vi "Run.vi"(8 "error in (no error)":errorcluster, 9 "s on last turn":dbl, 10 "Maze (0: Empty, -1: Enemy. >0: Teammate":i32[][](array[numeric]), 11 "Spawn in":refnum<class "Spawn.lvclass">) -> (0 "error out":errorcluster, 1 "Direction":T1, 2 "Action":T2, 3 "Spawn out":refnum<class "Spawn.lvclass">, 4 "Replicated":refnum<class "Runner.lvclass">)   [LabVIEW 2014, in "Spawn.lvclass"]
uses:
  Spawn.lvclass
  Action Enum.ctl
  Direction Enum.ctl
  Runner.lvclass
  Spawn.lvclass/Spawn.ctl
  Attack/Attack.lvclass
  Attack/Attack.lvclass/Attack.ctl
  Attack/Write Deviation.vi
  Attack/Write Direction.vi
  Attack/Write Frequency.vi
  SquareBattle.lvclass
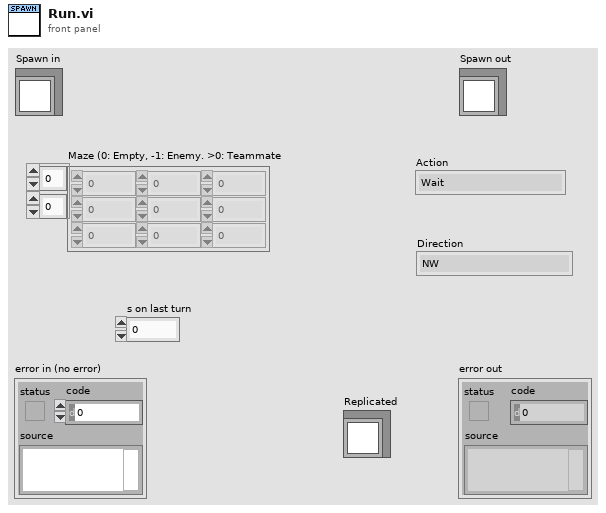
[diagram p1: front panel]
types:
  T1 = typedef "SquareBattle.lvclass/Direction Enum.ctl" = enum16{"NW", "N", "NE", "E", "SE", "S", "SW", "W"}
  T2 = typedef "SquareBattle.lvclass/Action Enum.ctl" = enum16{"Wait", "Move", "Attack", "Replicate"}
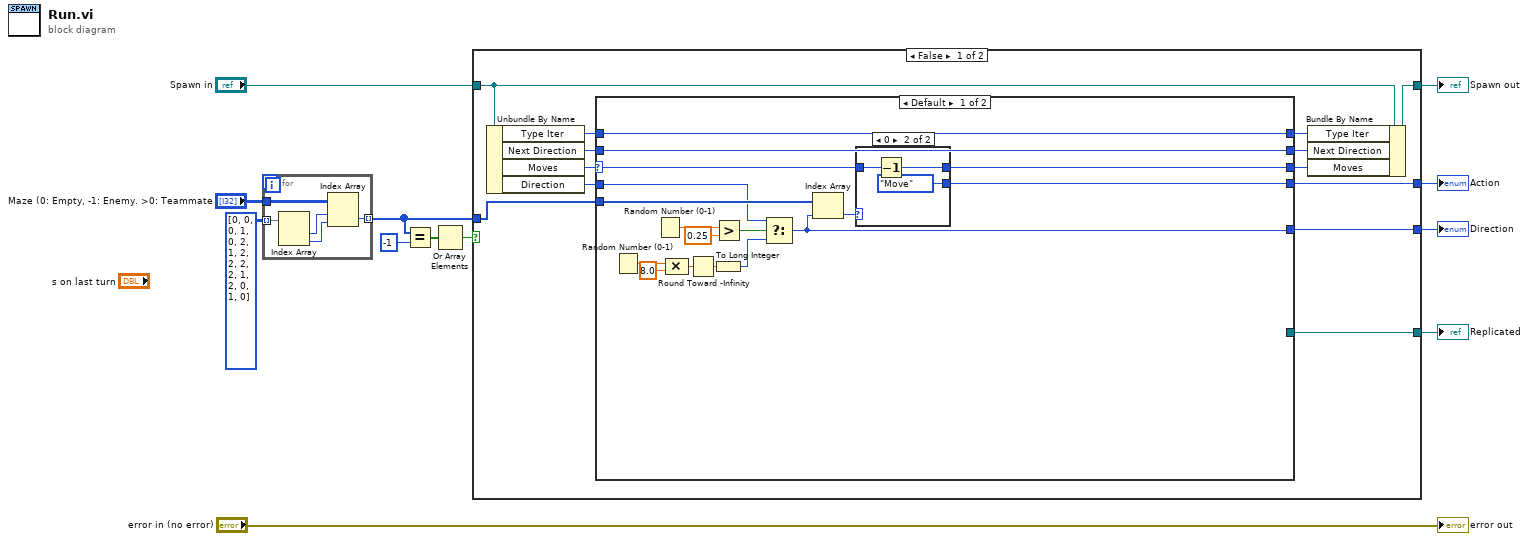
[diagram p0: block diagram]
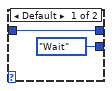
[diagram p2: hidden frame]
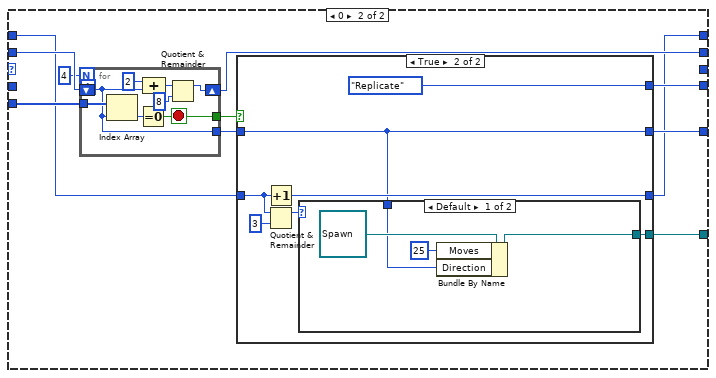
[diagram p3: hidden frame]
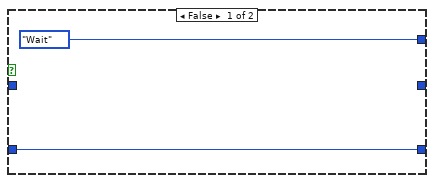
[diagram p4: hidden frame]
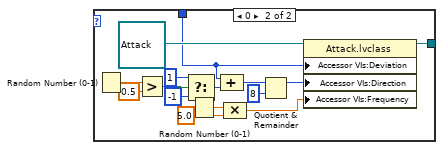
[diagram p5: hidden frame]
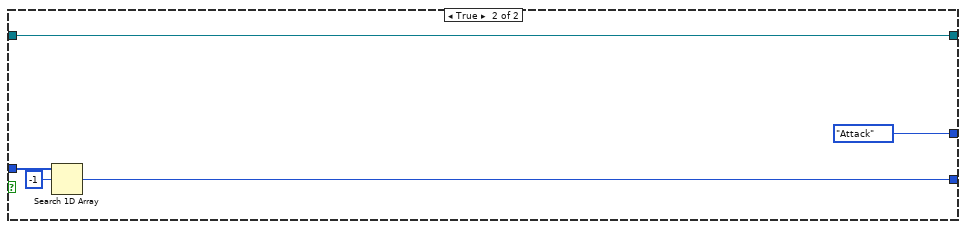
[diagram p6: hidden frame]
diagram:
  n1 = for {
    tunnel: "Maze (0: Empty, -1: Enemy. >0: Teammate" -> [w17]
    tunnel: i32[][] [[0, 0], [0, 1], [0, 2], [1, 2], [2, 2], [2, 1], [2, 0], [1, 0]] -> [w16] mode=indexing
    tunnel: [w13] -> w3 mode=indexing
    n2 = Index Array(array=w16) -> (element #1=w15:i32, element #2=w14:i32)  [unwired: 2 in]
    n3 = Index Array(array=w17, index (row)=w15, index (col)=w14) -> (element=w13:i32)
  }
  n4 = Equal?(x=w3, y=-1) -> (x = y?=w2:bool[])
  n5 = Or Array Elements(Boolean array=w2) -> (logical OR=w1:bool)
  n6 = case shown="False" w1 {
    tunnel: [w30 Action_Enum."Attack" ("Action")] -> w11
    tunnel: "Spawn in" -> [w28 w104]
    tunnel: [w27 w104] -> w9
    tunnel: [w25 w100] -> w8
    tunnel: [w23 _] -> w7
    tunnel: w3 -> [w20 w102]
    frame False {
      n7 = Unbundle By Name(w28) -> ("Type Iter"=w19:i32, "Next Direction"=w22:T1, "Moves"=w29:i32, "Direction"=w24:T1)
      n8 = case shown="Default" w29 {
        selector: w29 -> [w47 _]
        tunnel: [w45 w63] -> w30
        tunnel: [w46 _] -> w26
        tunnel: w24 -> [w32 _]
        tunnel: [w31 w62] -> w25
        tunnel: [_ w61] -> w23
        tunnel: w22 -> [w43 w60]
        tunnel: [w43 w59] -> w21
        tunnel: w20 -> [w42 w58]
        tunnel: w19 -> [w41 w57]
        tunnel: [w41 w56] -> w18
        frame Default {
          n9 = Random Number (0-1)() -> (number: 0 to 1=w38:dbl)
          n10 = Random Number (0-1)() -> (number: 0 to 1=w40:dbl)
          n11 = Compound Arithmetic op=MULTIPLY(w38, 8.0 ("value")) -> (w36:dbl)
          n12 = Round Toward -Infinity(1:w36) -> (0:w34:dbl)
          n13 = To Long Integer(number=w34) -> (32bit integer=w33:i32)
          n14 = Greater?(x=w40, y=0.25) -> (0:w35:bool)
          n15 = Select(t=w32, s=w35, f=w33) -> (s? t:f=w31:i32)
          n16 = Index Array(array=w42, index=w31) -> (element=w44:i32)
          n17 = case shown="0" w44 {
            tunnel: w47 -> [w49 w52]
            tunnel: [w49 w51] -> w46
            tunnel: [Action_Enum."Wait" ("Action") Action_Enum."Move" ("Action")] -> w45
            frame Default {
            }
            frame 0 {
              n18 = Decrement(x=w52) -> (x-1=w51:i32)
            }
          }
        }
        frame 0 {
          n19 = for {
            N: 4 -> [_]
            tunnel: w58 -> [w99]
            tunnel: [w97] -> w54
            shift-right: [w94] -> w59
            shift-left: w60 -> [w92]
            tunnel: [w92] -> w53
            stop <- w97 stop-if-true
            n20 = Index Array(array=w99, index=w92) -> (element=w98:i32)
            n21 = Equal To 0?(x=w98) -> (x = 0?=w97:bool)
            n22 = Compound Arithmetic op=ADD(2, w92) -> (w95:i32)
            n23 = Quotient & Remainder(x=w95, y=8) -> (x-y*floor(x/y)=w94:i32)  [unwired: 1 out]
          }
          n24 = case shown="True" w54 {
            tunnel: [Action_Enum."Wait" ("Action") Action_Enum."Replicate" ("Action")] -> w63
            tunnel: [_ w66] -> w62
            tunnel: w53 -> [_ w66]
            tunnel: w57 -> [w64 w70]
            tunnel: [w64 w69] -> w56
            tunnel: [_ w67] -> w61
            frame False {
            }
            frame True {
              n25 = Increment(x=w70) -> (x+1=w69:i32)
              n26 = Quotient & Remainder(x=w70, y=3) -> (x-y*floor(x/y)=w68:i32)  [unwired: 1 out]
              n27 = case shown="Default" w68 {
                tunnel: [w75 w90] -> w67
                tunnel: w66 -> [w73 w86]
                frame Default {
                  n28 = Bundle By Name(cluster=refnum<class "Spawn.lvclass"> refnum ("Spawn.lvclass"), "Moves"=25, "Direction"=w73) -> (w75:refnum<class "Spawn.lvclass">)
                }
                frame 0 {
                  n29 = Random Number (0-1)() -> (number: 0 to 1=w89:dbl)
                  n30 = Greater?(x=w89, y=0.5) -> (0:w87:bool)
                  n31 = Select(t=1, s=w87, f=-1) -> (s? t:f=w85:i32)
                  n32 = Random Number (0-1)() -> (number: 0 to 1=w79:dbl)
                  n33 = Compound Arithmetic op=ADD(w86, w85) -> (w82:i32)
                  n34 = Compound Arithmetic op=MULTIPLY(w79, 5.0 ("value")) -> (w77:dbl)
                  n35 = Quotient & Remainder(x=w82, y=8) -> (x-y*floor(x/y)=w81:i32)  [unwired: 1 out]
                  n36 = property class="Attack.lvclass"(reference=refnum<class "Attack.lvclass"> refnum ("Attack.lvclass"), "Accessor VIs:Deviation"=w86, "Accessor VIs:Direction"=w81, "Accessor VIs:Frequency"=w77) -> (reference out=w90:refnum<class "Attack.lvclass">)  [unwired: 1 in, 1 out]
                }
              }
            }
          }
        }
      }
      n37 = Bundle By Name(cluster=w28, "Type Iter"=w18, "Next Direction"=w21, "Moves"=w26) -> (w27:refnum<class "Spawn.lvclass">)
    }
    frame True {
      n38 = Search 1D Array(1D array=w102, element=-1) -> (index of element=w100:i32)  [unwired: 1 in]
    }
  }
  "Spawn out" <- w9
  "Action" <- w11
  "Direction" <- w8
  "Replicated" <- w7
  "error out" <- "error in (no error)"
